vi "RapidOX.vi"() -> ()   [LabVIEW 2013]
uses:
  <vilib>/Instr/_visa.llb/VISA Configure Serial Port (Instr).vi
panel:
  out "Engineering string":string
  out "O2 Concentration (%)":dbl
  in  "stop":bool
  out "error out":errorcluster
  in  "RapidOX":bool
  out "Waveform Chart 5":cluster{dbl}(graph)
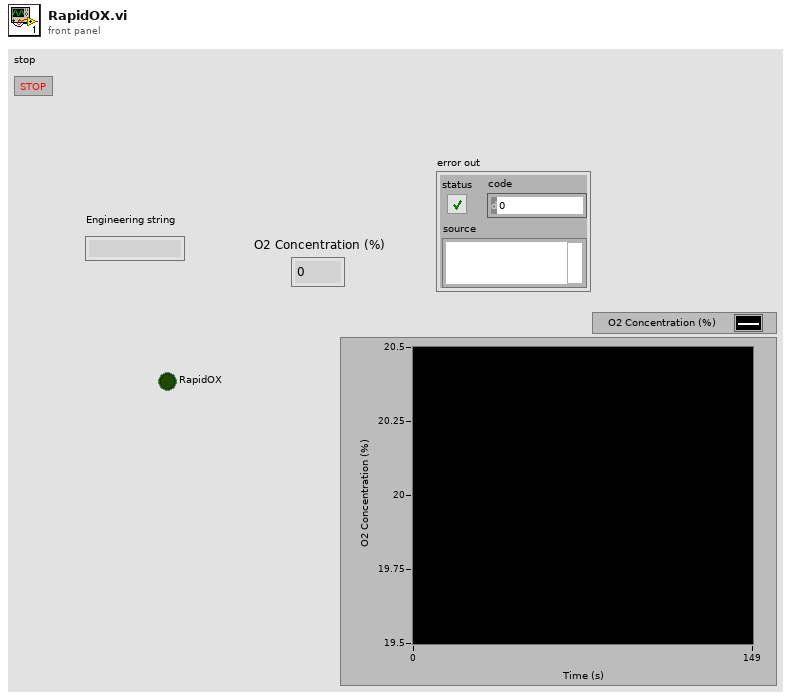
[diagram p1: front panel]
types:
  T1 = cluster{bool, "VISA resource name":refnum<visa-resource-name>, "error out":errorcluster}
  T2 = cluster{bool, "VISA resource name out":refnum<visa-resource-name>, "error out":errorcluster}
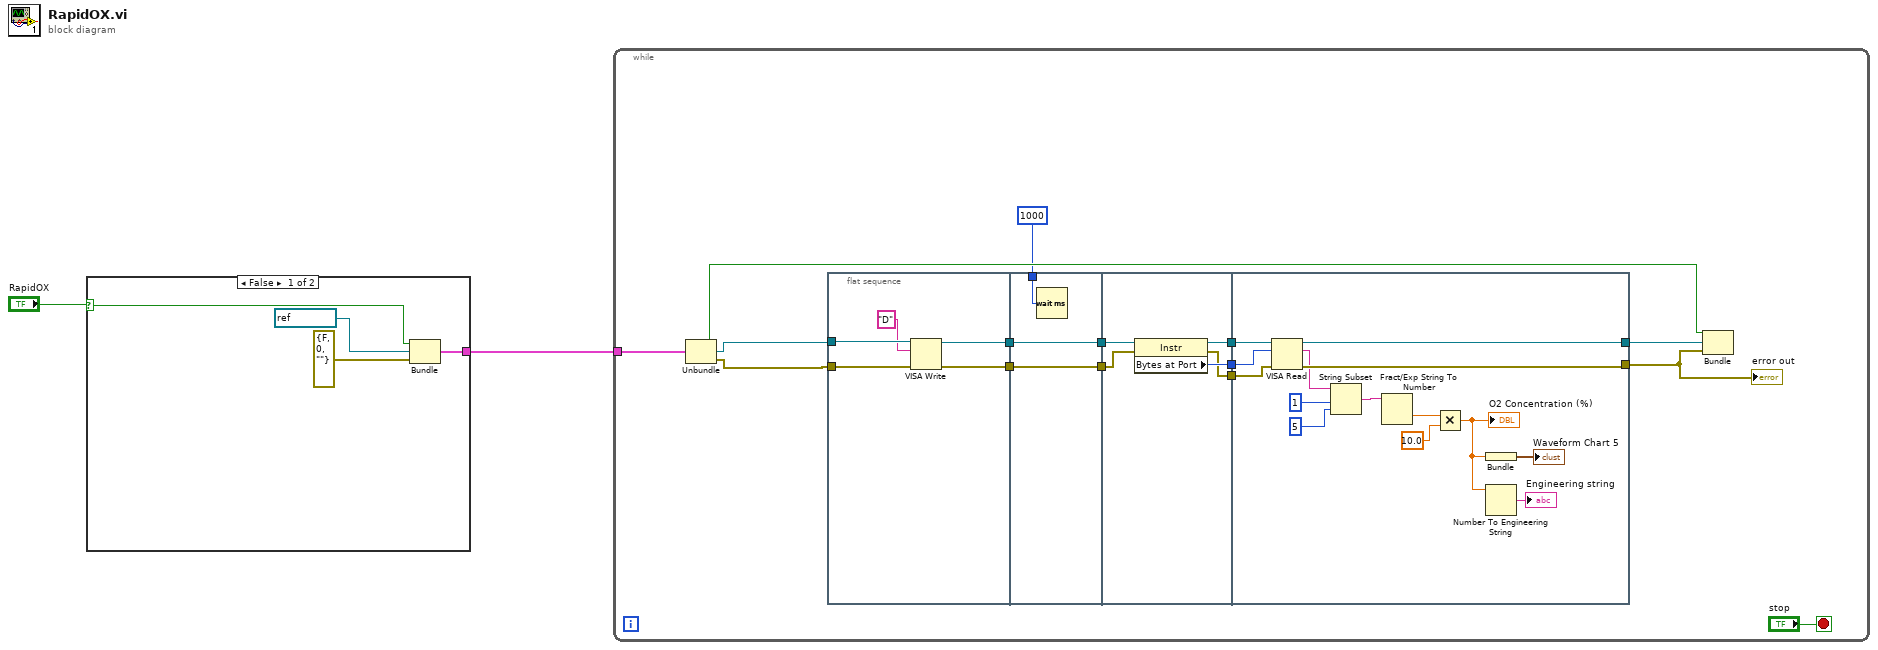
[diagram p0: block diagram]
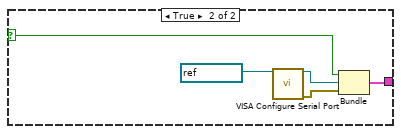
[diagram p2: hidden frame]
diagram:
  n1 = case shown="False" "RapidOX" {
    selector: "RapidOX" -> [w3 w7]
    tunnel: [w4 w8] -> w1
    frame False {
      n2 = Bundle(w3, "VISA resource name"=refnum<visa-resource-name> "COM7", "error out"=errorcluster {"status"=FALSE, "code"=0, "source"=""}) -> (w4:T1)  [unwired: 1 in]
    }
    frame True {
      n3 = call-poly "VISA Configure Serial Port"("VISA resource name"=refnum<visa-resource-name> "COM7") -> ("VISA resource name out"=w10:refnum<visa-resource-name>, "error out"=w9:errorcluster)  [unwired: 13 in]
      n4 = Bundle(w7, "VISA resource name out"=w10, "error out"=w9) -> (w8:T2)  [unwired: 1 in]
    }
  }
  n5 = while {
    tunnel: w1 -> [w19]
    stop <- "stop" stop-if-true
    n6 = Unbundle(w19) -> (w16:bool, "VISA resource name out"=w18:refnum<visa-resource-name>, "error out"=w17:errorcluster)
    n7 = flat-sequence {
      tunnel: w18 -> [w31]
      tunnel: w17 -> [w30]
      tunnel: [w28] -> w26
      tunnel: [w27] -> w25
      tunnel: [w34] -> w24
      tunnel: w26 -> [w34]
      tunnel: w25 -> [w33]
      tunnel: [w33] -> w23
      tunnel: u32 1000 ("milliseconds to wait") -> [w32]
      tunnel: w24 -> [w39]
      tunnel: w23 -> [w38]
      tunnel: [w37] -> w22
      tunnel: [w36] -> w21
      tunnel: [w35] -> w20
      tunnel: w22 -> [w53]
      tunnel: w21 -> [w52]
      tunnel: w20 -> [w51]
      tunnel: [w49] -> w14
      tunnel: [w50] -> w15
      frame #0 {
        n8 = VISA Write(VISA resource name=w31, write buffer="D", error in (no error)=w30) -> (VISA resource name out=w28:refnum<visa-resource-name>, error out=w27:errorcluster)  [unwired: 1 out]
      }
      frame #1 {
        n9 = Wait (ms)(milliseconds to wait=w32) -> ()  [unwired: 1 out]
      }
      frame #2 {
        n10 = property class="Instr"(reference=w39, error in=w38) -> (reference out=w37:refnum<visa-resource-name>, error out=w35:errorcluster, "Bytes at Port"=w36:u32)
      }
      frame #3 {
        n11 = VISA Read(VISA resource name=w53, byte count=w52, error in (no error)=w51) -> (VISA resource name out=w50:refnum<visa-resource-name>, read buffer=w48:string, error out=w49:errorcluster)  [unwired: 1 out]
        n12 = String Subset(string=w48, offset (0)=1, length (rest)=5 ("length (rest)")) -> (substring=w45:string)
        n13 = Fract/Exp String To Number(string=w45) -> (number=w43:dbl)  [unwired: 3 in, 1 out]
        n14 = Multiply(x=w43, y=10.0) -> (x*y=w40:dbl)
        "O2 Concentration (%)" <- w40
        n15 = Bundle(w40) -> (→"Waveform Chart 5":cluster{dbl})  [unwired: 1 in]
        n16 = Number To Engineering String(4:w40) -> (0:→"Engineering string":string)  [unwired: 3 in]
      }
    }
    n17 = Bundle(w16, "VISA resource name out"=w15, "error out"=w14) -> ()  [unwired: 1 in, 1 out]
    "error out" <- w14
  }
